vi "diode characteristic.vi"() -> ()   [LabVIEW 2018]
uses:
  <vilib>/Utility/file.llb/Read Delimited Spreadsheet (DBL).vi
panel:
  out "Prepared by \nthe project":string
  out "Diode Characteristic":dbl[](graph)
  in  "Measurement file \nwith extension Txt":path
  out "ID              VD":dbl[][](array[numeric])
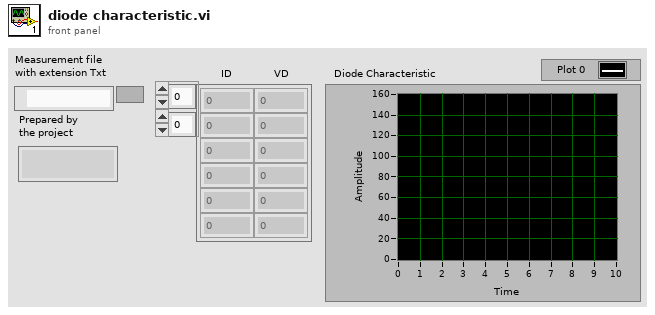
[diagram p1: front panel]
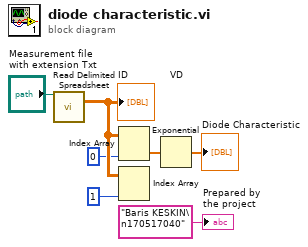
[diagram p0: block diagram]
diagram:
  n1 = call-poly <vilib>:"Read Delimited Spreadsheet.vi"("file path (dialog if empty)"="Measurement file \nwith extension Txt") -> ("all rows"=w6:dbl[][])  [unwired: 9 in, 5 out]
  "ID              VD" <- w6
  n2 = Index Array(array=w6, index (col)=0 ("disabled index (col)")) -> (element=w3:dbl[])  [unwired: 1 in]
  n3 = Index Array(array=w6, index (col)=1 ("disabled index (col)")) -> ()  [unwired: 1 in, 1 out]
  n4 = Exponential(1:w3) -> (0:→"Diode Characteristic":dbl[])
  "Prepared by \nthe project" <- "Baris KESKIN\n170517040"
